vi "globalUtilities.vi"() -> ()   [LabVIEW 2017]
panel:
  out "framesRead":u32
  in  "multiColorWormSettingsLaser":T1(array[cluster])=[{"laserWavelength (nm)"=405.0, "laserPower (mW)"=5.0, "sliderPosition"=0}, {"laserWavelength (nm)"=488.0, "laserPower (mW)"=20.0, "sliderPosition"=3}, {"laserWavelength (nm)"=561.0, "laserPower (mW)"=20.0, "sliderPosition"=1}]
  in  "multiColorWormSettings":T2(array[cluster])=[{"laserWavelength"=405.0, "exposureTime"=0.1, "filterWheelPosition"=1, "name"="BFP", "exposureTimeMultiplier"=1.0}, {"laserWavelength"=405.0, "exposureTime"=0.1, "filterWheelPosition"=2, "name"="Cerulean", "exposureTimeMultiplier"=1.0}, {"laserWavelength"=488.0, "exposureTime"=0.1, "filterWheelPosition"=3, "name"="GFP", "exposureTimeMultiplier"=1.0}, {"laserWavelength"=488.0, "exposureTime"=0.1, "filterWheelPosition"=4, "name"="mOrange", "exposureTimeMultiplier"=1.0}, {"laserWavelength"=561.0, "exposureTime"=0.1, "filterWheelPosition"=5, "name"="mCherry", "exposureTimeMultiplier"=1.0}, {"laserWavelength"=561.0, "exposureTime"=0.1, "filterWheelPosition"=6, "name"="mNeptune", "exposureTimeMultiplier"=1.0}, {"laserWavelength"=488.0, "exposureTime"=0.1, "filterWheelPosition"=5, "name"="CyOFP", "exposureTimeMultiplier"=1.0}]
  in  "multiColorWorm":bool
  out "framesSaved":u32
  out "volumesSaved":i32
  out "frameCurrentCount":i32
  out "frameCurrentIndex":i32
  out "volumeFirstFrameReferences":refnum<data-value>[](array[refnum])
  out "volumeDirectionReferences":refnum<data-value>[](array[refnum])
  out "frameBrightnessReferences":refnum<data-value>
  in  "acquisitionVolumeMaxN":i32=30000
  out "volumesAcquired":i32
  out "framesNotSaved":i32
  out "framesNotRead":i32
  out "acquisitionAutofocus":bool
  in  "acquisitionAsynchronousClock":u32=1
  out "fileAsynchronousError":errorcluster
  out "fileAsynchronousRefnum":refnum<file>
  out "fileBaseDiskAndFolder":string="D:\\Data\\"
  out "framesSaveLegacy":bool
  in  "daqAcquiring":bool
  in  "hamamatsuAcquiring":bool
  in  "mainStopped":bool
  in  "daqStop":bool
  in  "pharosPulseInterval":i32=1 min=1
  in  "pharosNPulses":i32 min=0
  out "acquisitionStart":bool
  in  "pharosTimeBeforeTriggering":u32=100
  in  "daqSave":bool
  in  "acquisitionStop":bool
  in  "acquisitionGuiUpdateDivider":i32=16
  out "framesTickcountOfFirstSaved":u32
  out "framesIndexOfFirstSaved":i32
  out "framesTimestampOfFirstSaved":dbl
  in  "framesSave":bool
  out "filesFolderName":string
  in  "acquisitionFramesPerSecond":dbl=100.0
  in  "acquisitionVolumeHeight":dbl=50.0
  in  "acquisitionVolumesPerSecond":dbl=3.0
  in  "generalStop":bool
  # "SOFTWARE"
  # "ACQUISITION \nPARAMETERS"
  # "FILE STORAGE"
  # "VOLUMES"
  # "MULTICOLOR WORM"
  # "FRAMES"
  # "um"
  # "ms"
  # "405 0\nGfp 3\nmcherry 1"
  # "OPTOGENETICS"
  # "ms"
  # "(1/rep rate)"
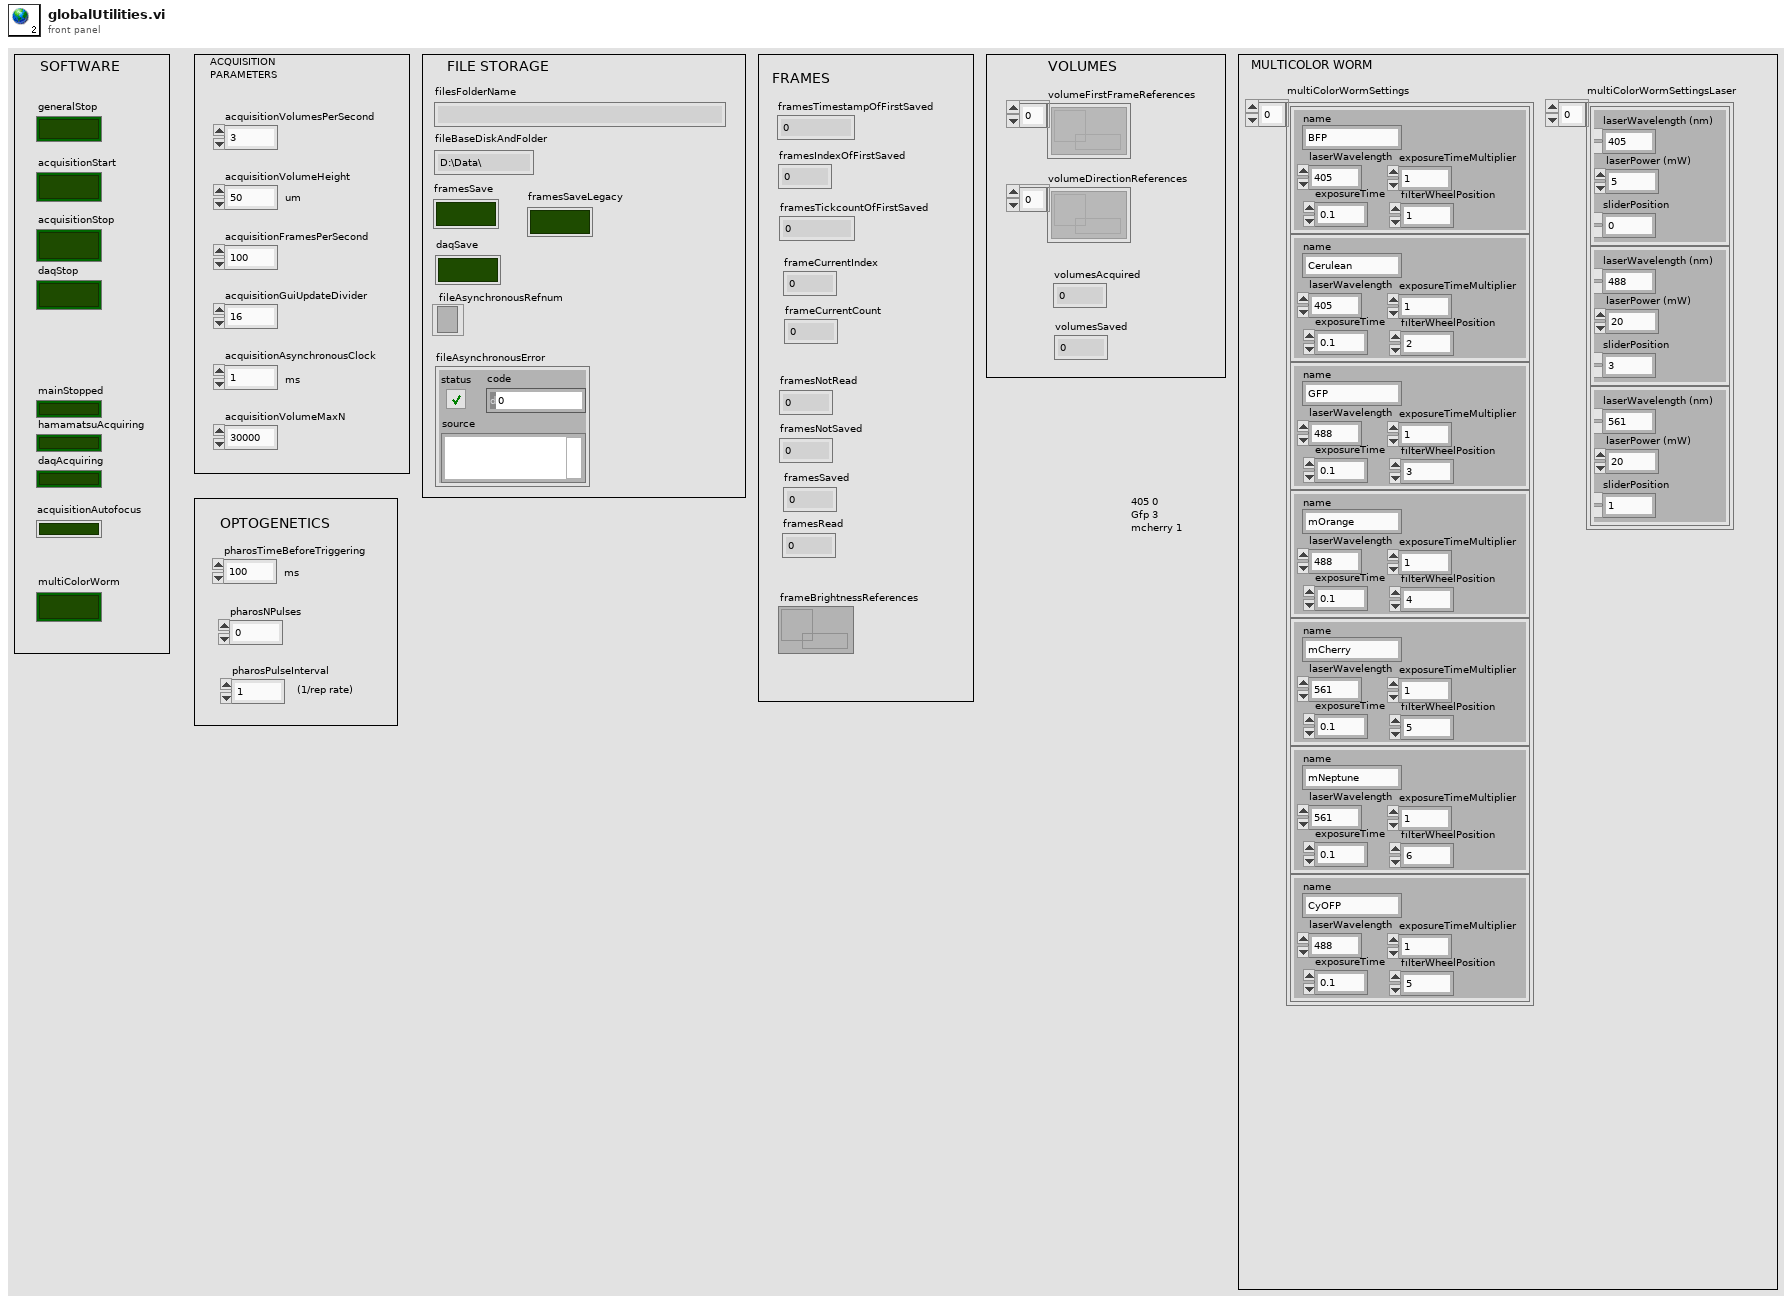
[diagram p1: front panel]
types:
  T1 = cluster{"laserWavelength (nm)":dbl, "laserPower (mW)":dbl, "sliderPosition":i32}[]
  T2 = cluster{"laserWavelength":dbl, "exposureTime":dbl, "filterWheelPosition":i32, "name":string, "exposureTimeMultiplier":dbl}[]
diagram:
